vi "Users_IDs_from_string.vi"(8 "error in":errorcluster, 11 "input string":string="[11] [2] [3]") -> (0 "error out":errorcluster, 2 "Preformed string":string, 3 "Users_ID_from_string":string[](array[string]))   [LabVIEW 2015, in "DB.lvclass"]
uses:
  DB.lvclass
  <vilib>/regexp/Match Regular Expression.xnode
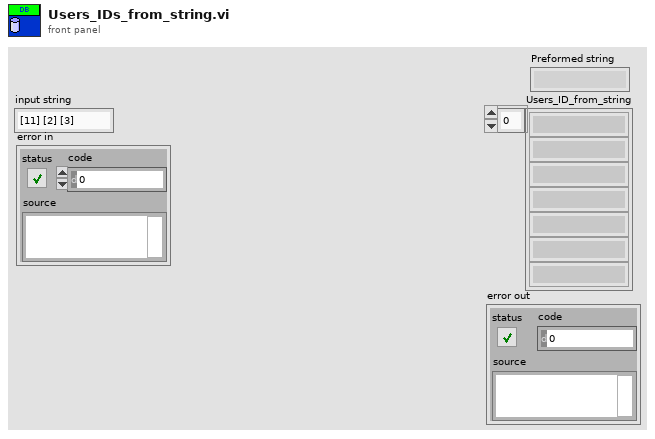
[diagram p1: front panel]
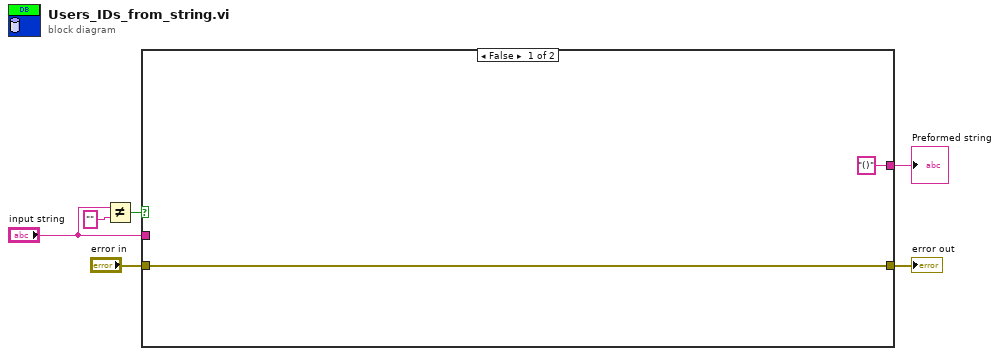
[diagram p0: block diagram]
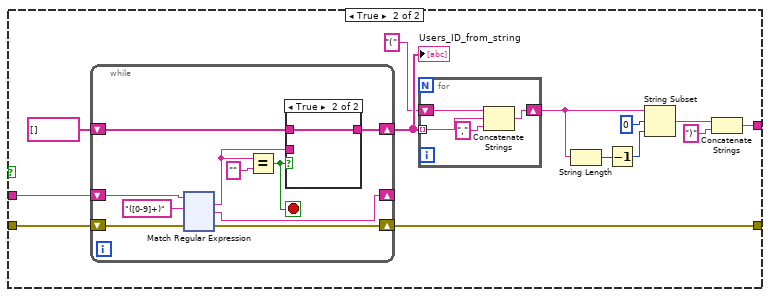
[diagram p2: hidden frame]
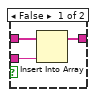
[diagram p3: hidden frame]
diagram:
  n1 = Not Equal?(x="input string", y="") -> (x != y?=w1:bool)
  n2 = case shown="False" w1 {
    tunnel: "error in" -> [w7 w20]
    tunnel: [w7 w19] -> w5
    tunnel: ["()" w10] -> w4
    tunnel: "input string" -> [_ w9]
    frame False {
    }
    frame True {
      n3 = while {
        shift-right: [w34] -> _
        shift-left: w9 -> [w35]
        shift-right: [w29] -> w18
        shift-left: string[] [] ("Array") -> [w28]
        shift-right: [w26] -> w19
        shift-left: w20 -> [w27]
        stop <- w30 stop-if-true
        n4 = xnode "Match Regular Expression"("input string"=w35, "regular expression"="([0-9]+)", "error in"=w27) -> ("whole match"=w32:string, "after match"=w34:string, "error out"=w26:errorcluster)  [unwired: 3 in, 2 out]
        n5 = Equal?(x=w32, y="") -> (x = y?=w30:bool)
        n6 = case shown="True" w30 {
          tunnel: w32 -> [w38 _]
          tunnel: [w36 w39] -> w29
          tunnel: w28 -> [w37 w39]
          frame False {
            n7 = Insert Into Array(array=w37, new element=w38) -> (w36:string[])  [unwired: 1 in]
          }
          frame True {
          }
        }
      }
      "Users_ID_from_string" <- w18
      n8 = for {
        tunnel: w18 -> [w25] mode=indexing
        shift-right: [w22] -> w15
        shift-left: "(" -> [w24]
        n9 = Concatenate Strings(w24, w25, "," ("string")) -> (w22:string)
      }
      n10 = String Length(string=w15) -> (length=w14:i32)
      n11 = Decrement(x=w14) -> (x-1=w13:i32)
      n12 = String Subset(string=w15, offset (0)=0, length (rest)=w13) -> (substring=w12:string)
      n13 = Concatenate Strings(w12, ")" ("string")) -> (w10:string)
    }
  }
  "error out" <- w5
  "Preformed string" <- w4
